vi "Query Output Safety.vi"(0 "VISA resource name":refnum<visa-resource-name>, 11 "error in (no error)":errorcluster) -> (4 "VISA resource name out":refnum<visa-resource-name>, 6 "Output Safety":T1, 15 "error out":errorcluster)   [LabVIEW 2012, in "NH Research Regenerative Test Series.lvlib"]
doc: "Returns the maximum allowable time and value, which, if exceeded, will cause the Module to shut off. Time values of <0 indicate that parameter is disabled."
uses:
  <instrlib>/NH Research Regenerative Test Series/NH Research Regenerative Test Series.lvlib
  <instrlib>/NH Research Regenerative Test Series/Public/Configure/Output Safety.ctl
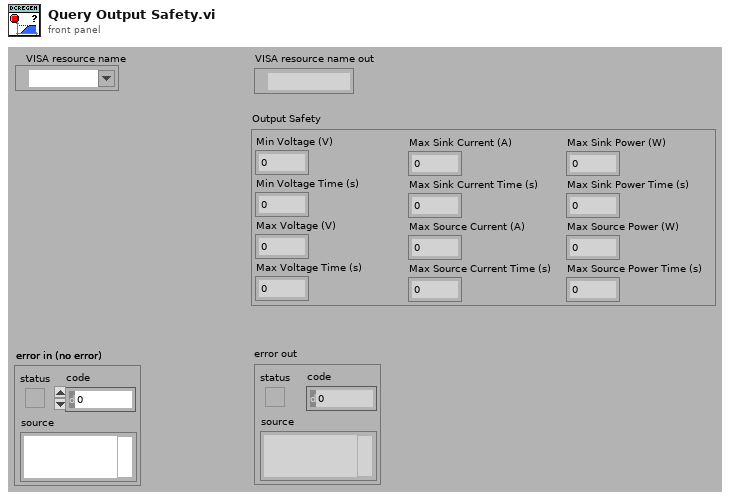
[diagram p1: front panel]
types:
  T1 = typedef "NH Research Regenerative Test Series.lvlib/Output Safety.ctl" = cluster{"Min Voltage (V)":dbl, "Min Voltage Time (s)":dbl, "Max Voltage (V)":dbl, "Max Voltage Time (s)":dbl, "Max Sink Current (A)":dbl, "Max Sink Current Time (s)":dbl, "Max Source Current (A)":dbl, "Max Source Current Time (s)":dbl, "Max Sink Power (W)":dbl, "Max Sink Power Time (s)":dbl, "Max Source Power (W)":dbl, "Max Source Power Time (s)":dbl}
  T2 = cluster{"[0]":dbl, "[1]":dbl, "[2]":dbl, "[3]":dbl, "[4]":dbl, "[5]":dbl, "[6]":dbl, "[7]":dbl, "[8]":dbl, "[9]":dbl, "[10]":dbl, "[11]":dbl}
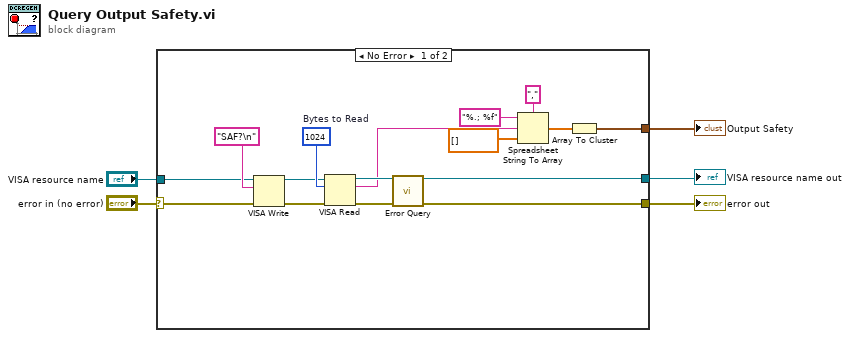
[diagram p0: block diagram]
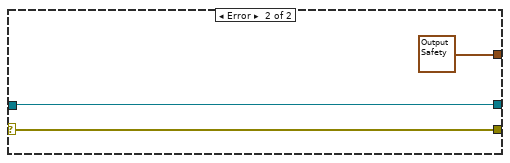
[diagram p2: hidden frame]
diagram:
  n1 = case shown="No Error" "error in (no error)" {
    selector: "error in (no error)" -> [w17 w24]
    tunnel: [w6 w24] -> w4
    tunnel: [w15 w23] -> w2
    tunnel: "VISA resource name" -> [w16 w23]
    tunnel: [w7 T1 {"Min Voltage (V)"=0.0, "Min Voltage Time (s)"=0.0, "Max Voltage (V)"=0.0, "Max Voltage Time (s)"=0.0, "Max Sink Current (A)"=0.0, "Max Sink Current Time (s)"=0.0, "Max Source Current (A)"=0.0, "Max Source Current Time (s)"=0.0, "Max Sink Power (W)"=0.0, "Max Sink Power Time (s)"=0.0, "Max Source Power (W)"=0.0, "Max Source Power Time (s)"=0.0} ("Output Safety")] -> w1
    frame No Error {
      w21 = u32 1024  # Bytes to Read
      n2 = VISA Write(VISA resource name=w16, write buffer="SAF?\n", error in (no error)=w17) -> (VISA resource name out=w19:refnum<visa-resource-name>, error out=w20:errorcluster)  [unwired: 1 out]
      n3 = VISA Read(VISA resource name=w19, byte count=w21, error in (no error)=w20) -> (VISA resource name out=w14:refnum<visa-resource-name>, read buffer=w8:string, error out=w13:errorcluster)  [unwired: 1 out]
      n4 = call <instrlib>:"Error Query.vi"("VISA resource name"=w14, "error in (no error)"=w13) -> ("VISA resource name out"=w15:refnum<visa-resource-name>, "error out"=w6:errorcluster)  [unwired: 10 in, 2 out]
      n5 = Spreadsheet String To Array(delimiter (Tab)=",", format string="%.; %f", spreadsheet string=w8, array type (2D Dbl)=dbl[] []) -> (array=w9:dbl[])
      n6 = Array To Cluster(array=w9) -> (cluster=w7:T2)
    }
    frame Error {
    }
  }
  "error out" <- w4
  "VISA resource name out" <- w2
  "Output Safety" <- w1
